vi "Deterministic Errors.New Allocated String (16B).vi"() -> (3 "16-byte string":string)   [LabVIEW 2016, in "Deterministic Error Builder.lvlib"]
uses:
  Deterministic Error Builder.lvlib
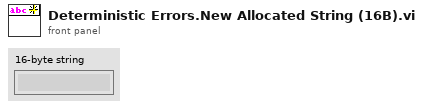
[diagram p1: front panel]
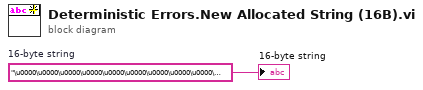
[diagram p0: block diagram]
diagram:
  w1 = "\u0000\u0000\u0000\u0000\u0000\u0000\u0000\u0000\u0000\u0000\u0000\u0000\u0000\u0000\u0000\u0000"  # 16-byte string
  "16-byte string" <- w1
